vi "Test Process Log Handler Configured.vi"(8 "error in (no error)":errorcluster, 11 "Process Test In":refnum<class "Process Test.lvclass">) -> (0 "error out":errorcluster, 3 "Process Test Out":refnum<class "Process Test.lvclass">)   [LabVIEW 2020, in "Process Test.lvclass"]
uses:
  Process Test.lvclass
  Process Test.lvclass/Process Test.ctl
  Framework/Process/Process.lvclass
  Mock Log Handler/Mock Log Handler.lvclass
  <vilib>/Astemes/LUnit/Test Case.lvclass
  C:/Git/astemes-triarc-framework/source/Framework/Base/Base.lvclass
  C:/Git/astemes-triarc-framework/source/Framework Test Suite/Mock Log Handler/Mock Log Handler.lvclass
  C:/Git/astemes-triarc-framework/source/Framework/Logging/Logging.lvclass
  C:/Git/astemes-triarc-framework/source/Framework Test Suite/Base Class Test/Base Test.lvclass
  C:/Program Files (x86)/National Instruments/LabVIEW 2020/vi.lib/Astemes/LUnit/Test Case.lvclass
  C:/Git/astemes-triarc-framework/source/Framework Test Suite/Process Test/Process Test.lvclass
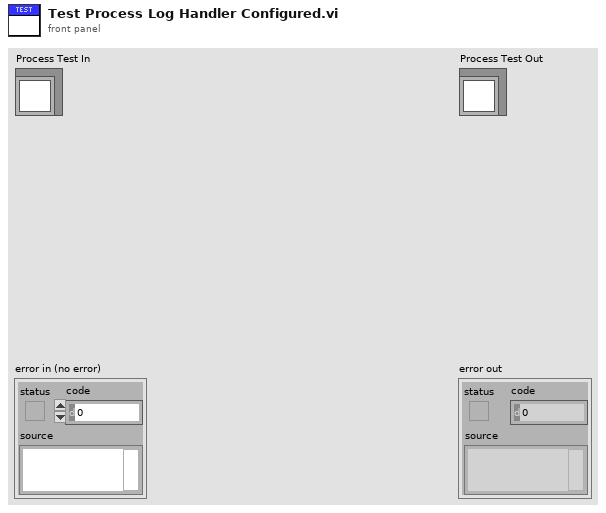
[diagram p1: front panel]
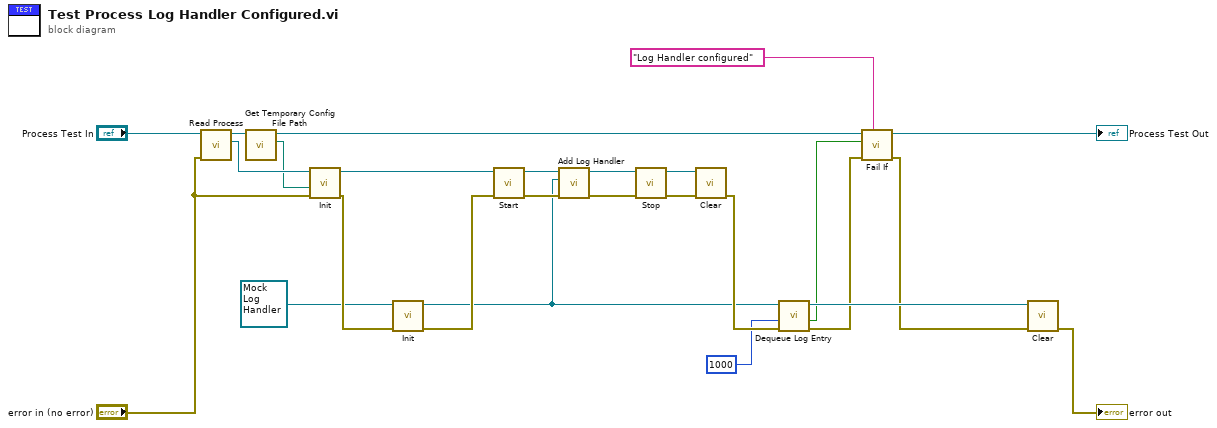
[diagram p0: block diagram]
diagram:
  n1 = call "Read Process.vi"("error in (no error)"="error in (no error)", "Process Test in"="Process Test In") -> ("Process.lvclass"=w14:refnum<class "Process.lvclass">, "Process Test out"=w3:refnum<class "Process Test.lvclass">)  [unwired: 7 in, 1 out]
  n2 = call "Get Temporary Config File Path.vi"("Base Test in"=w3) -> ("Temporary Config File Path"=w1:path, "Base Test out"=w2:refnum<class "Process Test.lvclass">)  [unwired: 8 in, 1 out]
  n3 = call-dynamic "Init.vi"("error in (no error)"="error in (no error)", "Config File Path"=w1, "Process In"=w14) -> ("error out"=w25:errorcluster, "Process Out"=w6:refnum<class "Process.lvclass">)  [unwired: 7 in]
  n4 = call-dynamic "Init.vi"("error in (no error)"=w25, "Mock Log Handler In"=refnum<class "Mock Log Handler.lvclass"> refnum ("Mock Log Handler.lvclass")) -> ("error out"=w21:errorcluster, "Mock Log Handler Out"=w4:refnum<class "Mock Log Handler.lvclass">)  [unwired: 8 in]
  n5 = call "Start.vi"("error in (no error)"=w21, "Process In"=w6) -> ("error out"=w7:errorcluster, "Process Out"=w5:refnum<class "Process.lvclass">)  [unwired: 7 in, 1 out]
  n6 = call "Add Log Handler.vi"("error in (no error)"=w7, "Log Handler"=w4, "Process In"=w5) -> ("error out"=w22:errorcluster, "Process Out"=w23:refnum<class "Process.lvclass">)  [unwired: 7 in]
  n7 = call "Stop.vi"("error in (no error)"=w22, "Process In"=w23) -> ("error out"=w9:errorcluster, "Process Out"=w8:refnum<class "Process.lvclass">)  [unwired: 7 in, 1 out]
  n8 = call-dynamic "Clear.vi"("error in (no error)"=w9, "Process In"=w8) -> ("error out"=w18:errorcluster)  [unwired: 9 in]
  n9 = call "Dequeue Log Entry.vi"("error in (no error)"=w18, "timeout in ms (-1)"=1000, "Mock Log Handler in"=w4) -> ("error out"=w17:errorcluster, "timed out?"=w10:bool, "Mock Log Handler out"=w20:refnum<class "Mock Log Handler.lvclass">)  [unwired: 5 in, 1 out]
  n10 = call <vilib>:"Fail If.vi"("Description"="Log Handler configured", "error in (no error)"=w17, "Fail?"=w10, "LUnit Test Case In"=w2) -> ("error out"=w16:errorcluster, "LUnit Test Case Out"=→"Process Test Out":refnum<class "Process Test.lvclass">)  [unwired: 6 in]
  n11 = call-dynamic "Clear.vi"("error in (no error)"=w16, "Mock Log Handler In"=w20) -> ("error out"=→"error out":errorcluster)  [unwired: 9 in]
